vi "control_Indication.vi"(7 "Параметры":T1, 8 "Error In":errorcluster, 9 "control_Pair ref in":refnum<vi>, 10 "control_Port_2 ref in":refnum<vi>, 11 "control_Port_1 ref in":refnum<vi>) -> (0 "Error Out":errorcluster, 1 "control_Pair ref out":refnum<vi>, 2 "control_Port_2 ref out":refnum<vi>, 3 "control_Port_1 ref out":refnum<vi>)   [LabVIEW 2023, in "pump_Lib.lvlib"]
uses:
  pump_Lib.lvlib
  TypeDef/pump_Type.ctl
  TypeDef/pair_Type.ctl
  TypeDef/parametrs_Type.ctl
panel:
  # "%"
  # "%"
  # "%"
  # "%"
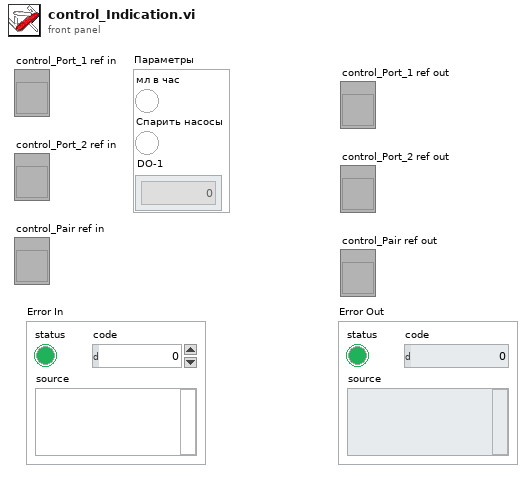
[diagram p1: front panel]
types:
  T1 = typedef "pump_Lib.lvlib/parametrs_Type.ctl" = cluster{"мл в час":bool, "Спарить насосы":bool, "DO-1":u16[]}
  T2 = enum8{"Enabled", "Disabled", "Disabled and Grayed Out"}
  T3 = typedef "pump_Lib.lvlib/pump_Type.ctl" = cluster{"Давление заданное":dbl, "Давление MAX заданное":dbl, "Давление в насосе":dbl, "Давление в системе":dbl, "Расход заданый":dbl, "Расход текущий":dbl, "Объём заданный":dbl, "Объём текущий":dbl, "Позиция насоса %":dbl, "Ток двигателя":dbl, "controlMsg":string, "Клапан k_sys":bool, "Клапан k_res":bool, "Клапан k_air":bool, "Вверх":bool, "Домой":bool, "Вниз":bool, "Старт расход":bool, "Старт давление":bool, "Сброс объёма":bool, "Сброс давления Рсис":bool, "Сброс давления Рнас":bool, "Bits":cluster{"plc_control":bool, "lag_control":bool, "mstop_control":bool, "st_home":bool, "error":bool, "mstart":bool, "pair":bool, "startQ":bool, "startP":bool, "volume_Stop":bool}}
  T4 = typedef "pump_Lib.lvlib/pair_Type.ctl" = cluster{"Давление заданное":dbl, "Давление в системе":dbl, "Расход заданый":dbl, "Расход текущий":dbl, "Объём заданный":dbl, "Объём текущий":dbl, "Старт давление":bool, "Старт расход":bool, "Сброс объёма":bool, "plc_control":bool, "lag_control":bool, "mstop_control":bool, "Давление":cluster{"АЦП CH 0":dbl, "АЦП CH 1":dbl, "АЦП CH 2":dbl, "АЦП CH 3":dbl, "АЦП CH 4":dbl, "АЦП CH 5":dbl, "АЦП CH 6":dbl, "АЦП CH 7":dbl}, "Modbus":cluster{"Массив чтения":u16[], "Массив записи":u16[]}}
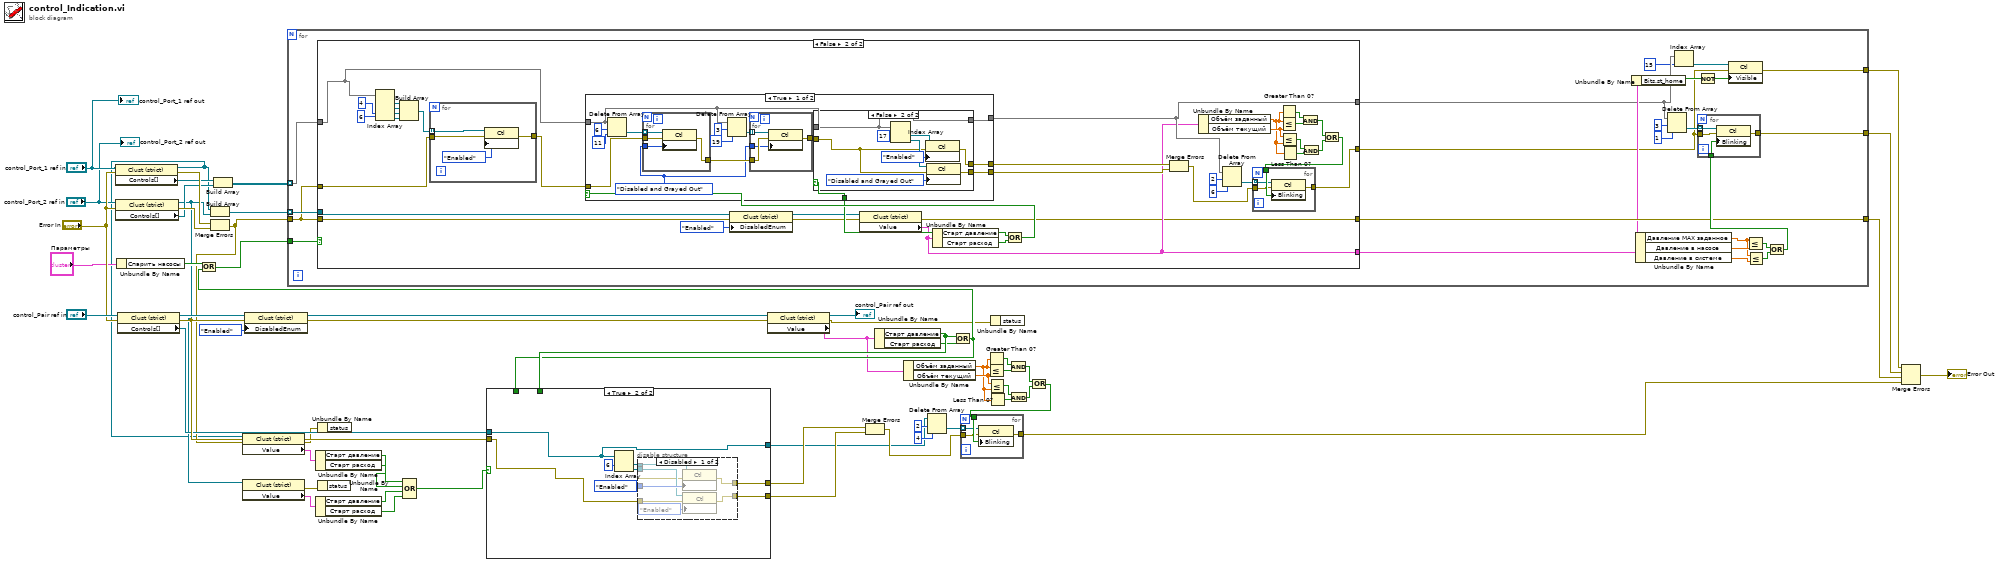
[diagram p0: block diagram]
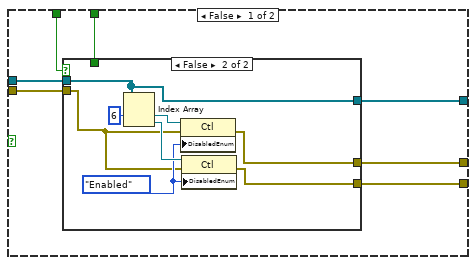
[diagram p2: hidden frame]
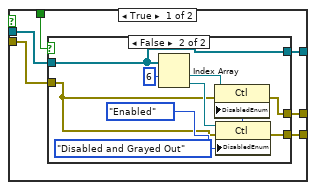
[diagram p3: hidden frame]
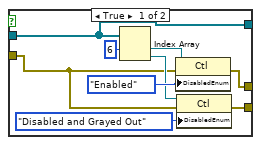
[diagram p4: hidden frame]
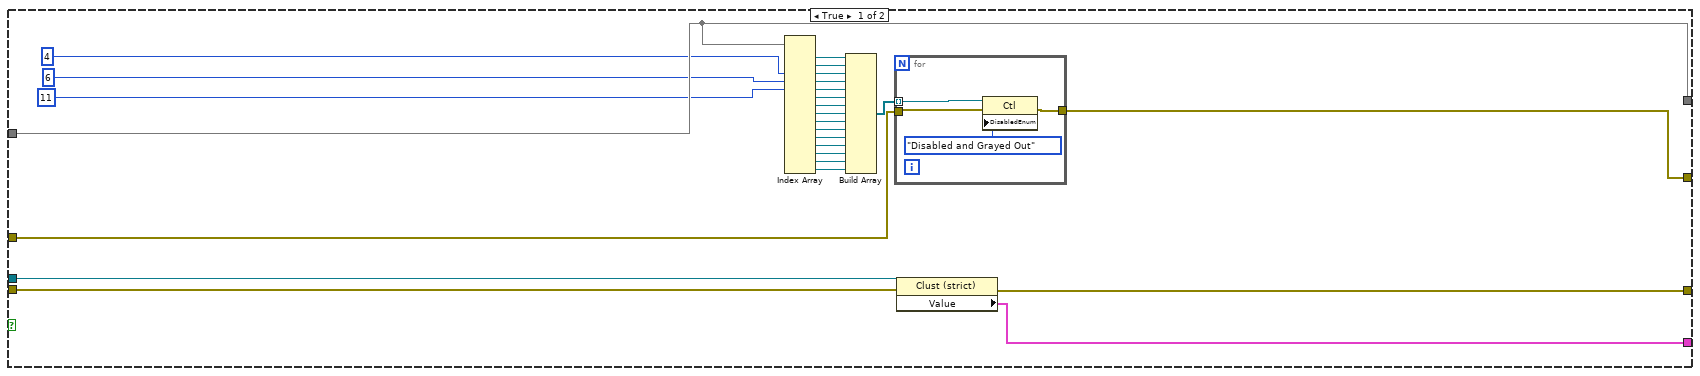
[diagram p6: hidden frame]
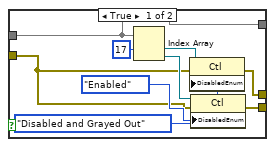
[diagram p7: hidden frame]
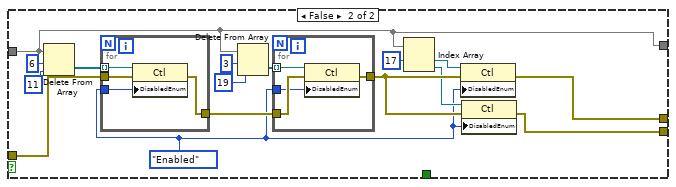
[diagram p8: hidden frame]
diagram:
  n1 = property class="Clust (strict)"(reference="control_Port_1 ref in", error in="Error In") -> (reference out=w11:refnum<vi>, error out=w55:errorcluster, "Controls[]"=w52:refnum<vi>[])
  n2 = property class="Clust (strict)"(reference="control_Port_2 ref in", error in="Error In") -> (reference out=w12:refnum<vi>, error out=w54:errorcluster, "Controls[]"=w51:refnum<vi>[])
  n3 = Unbundle By Name("Параметры") -> ("Спарить насосы"=w41:bool)
  n4 = property class="Clust (strict)"(reference="control_Pair ref in", error in="Error In") -> (reference out=w45:refnum<vi>, error out=w44:errorcluster, "Controls[]"=w43:refnum<vi>[])
  n5 = Build Array(w11, w12) -> (w53:refnum<vi>[])
  n6 = Merge Errors(w55, w54) -> (w13:errorcluster)
  n7 = Build Array(w52, w51) -> (w56:refnum<vi>[][])
  n8 = property class="Clust (strict)"(reference=w11, error in=w13) -> (error out=w8:errorcluster, "Value"=w10:T3)  [unwired: 1 out]
  n9 = property class="Clust (strict)"(reference=w12) -> (error out=w7:errorcluster, "Value"=w9:T3)  [unwired: 1 in, 1 out]
  n10 = property class="Clust (strict)"(reference=w45, error in=w44, "DisabledEnum"=T2."Enabled" ("Disabled")) -> (reference out=w47:refnum<vi>, error out=w48:errorcluster)
  n11 = Unbundle By Name(w10) -> ("Старт давление"=w6:bool, "Старт расход"=w5:bool)
  n12 = Unbundle By Name(w9) -> ("Старт давление"=w4:bool, "Старт расход"=w3:bool)
  n13 = Unbundle By Name(w7) -> ()  [unwired: 1 out]
  n14 = Unbundle By Name(w8) -> ()  [unwired: 1 out]
  n15 = Compound Arithmetic op=OR(w6, w5, w4, w3) -> (w2:bool)
  n16 = property class="Clust (strict)"(reference=w47, error in=w48) -> (reference out=→"control_Pair ref out":refnum<vi>, error out=w1:errorcluster, "Value"=w30:T4)
  n17 = Unbundle By Name(w30) -> ("Старт давление"=w50:bool, "Старт расход"=w49:bool)
  n18 = Unbundle By Name(w30) -> ("Объём заданный"=w26:dbl, "Объём текущий"=w27:dbl)
  n19 = Or(x=w50, y=w49) -> (x .or. y?=w39:bool)
  n20 = Or(x=w41, y=w39) -> (x .or. y?=w40:bool)
  n21 = for {
    tunnel: w56 -> [w81] mode=indexing
    tunnel: w53 -> [w80] mode=indexing
    tunnel: w13 -> [w79]
    tunnel: w40 -> [w78]
    tunnel: [w68] -> w16
    tunnel: [w67] -> w17
    tunnel: [w60] -> w14
    n22 = case shown="False" w78 {
      tunnel: w81 -> [w107 w130]
      tunnel: w79 -> [w87 w128]
      tunnel: w80 -> [w110 w118]
      tunnel: w79 -> [w111 w117]
      tunnel: [w107 w134] -> w64
      tunnel: [w86 w133] -> w61
      tunnel: [w109 w132] -> w66
      tunnel: [w108 w131] -> w68
      frame True {
        n23 = Index Array(array=w107, index #3=4 ("index"), index #4=6 ("index"), index #5=11 ("index")) -> (element #1=w103:refnum<vi>, element #2=w102:refnum<vi>, element #3=w101:refnum<vi>, element #4=w100:refnum<vi>, element #5=w99:refnum<vi>, element #6=w98:refnum<vi>, element #7=w97:refnum<vi>, element #8=w95:refnum<vi>, element #9=w96:refnum<vi>, element #10=w94:refnum<vi>, element #11=w93:refnum<vi>, element #12=w92:refnum<vi>, element #13=w91:refnum<vi>, element #14=w90:refnum<vi>, element #15=w89:refnum<vi>)  [unwired: 12 in]
        n24 = Build Array(w103, w102, w101, w100, w99, w98, w97, w95, w96, w94, w93, w92, w91, w90, w89) -> (w88:refnum<vi>[])
        n25 = for {
          tunnel: w88 -> [w115] mode=indexing
          tunnel: w87 -> [w114]
          tunnel: [w113] -> w86
          n26 = property class="Ctl"(reference=w115, error in=w114, "DisabledEnum"=T2."Disabled and Grayed Out" ("Disabled")) -> (error out=w113:errorcluster)  [unwired: 1 out]
        }
        n27 = property class="Clust (strict)"(reference=w110, error in=w111) -> (error out=w108:errorcluster, "Value"=w109:T3)  [unwired: 1 out]
      }
      frame False {
        n28 = Index Array(array=w130, index #3=4 ("index"), index #4=6 ("index")) -> (element #1=w123:refnum<vi>, element #2=w124:refnum<vi>, element #3=w125:refnum<vi>, element #4=w126:refnum<vi>)  [unwired: 2 in]
        n29 = Build Array(w123, w124, w125, w126) -> (w127:refnum<vi>[])
        n30 = for {
          tunnel: w127 -> [w156] mode=indexing
          tunnel: w128 -> [w155]
          tunnel: [w154] -> w129
          n31 = property class="Ctl"(reference=w156, error in=w155, "DisabledEnum"=T2."Enabled" ("Disabled")) -> (error out=w154:errorcluster)  [unwired: 1 out]
        }
        n32 = property class="Clust (strict)"(reference=w118, error in=w117, "DisabledEnum"=T2."Enabled" ("Disabled")) -> (reference out=w119:refnum<vi>, error out=w120:errorcluster)
        n33 = property class="Clust (strict)"(reference=w119, error in=w120) -> (error out=w131:errorcluster, "Value"=w132:T3)  [unwired: 1 out]
        n34 = Unbundle By Name(w132) -> ("Старт давление"=w150:bool, "Старт расход"=w152:bool)
        n35 = Or(x=w150, y=w152) -> (x .or. y?=w151:bool)
        n36 = case shown="True" w151 {
          tunnel: w129 -> [w172 w214]
          tunnel: w130 -> [w165 w204]
          tunnel: [w164 w204] -> w134
          tunnel: w150 -> [w163 _]
          tunnel: [w162 w203] -> w137
          tunnel: [w161 w202] -> w136
          frame True {
            w167 = T2."Disabled and Grayed Out" ("Disabled")
            n37 = Delete From Array(array=w165, length=6, index=11) -> (deleted portion=w173:refnum<vi>[])  [unwired: 1 out]
            n38 = for {
              tunnel: w173 -> [w201] mode=indexing
              tunnel: w172 -> [w200]
              tunnel: w167 -> [w199]
              tunnel: [w198] -> w168
              n39 = property class="Ctl"(reference=w201, error in=w200, "DisabledEnum"=w199) -> (error out=w198:errorcluster)  [unwired: 1 out]
            }
            n40 = Delete From Array(array=w165, length=3, index=19) -> (deleted portion=w169:refnum<vi>[])  [unwired: 1 out]
            n41 = for {
              tunnel: w169 -> [w197] mode=indexing
              tunnel: w168 -> [w196]
              tunnel: w167 -> [w195]
              tunnel: [w194] -> w166
              n42 = property class="Ctl"(reference=w197, error in=w196, "DisabledEnum"=w195) -> (error out=w194:errorcluster)  [unwired: 1 out]
            }
            n43 = case shown="False" w163 {
              tunnel: w165 -> [w179 w187]
              tunnel: [w179 w187] -> w164
              tunnel: w166 -> [w178 w188]
              tunnel: [w177 w186] -> w162
              tunnel: [w176 w185] -> w161
              frame True {
                n44 = Index Array(array=w179, index #1=17 ("index")) -> (element #1=w183:refnum<vi>, element #2=w182:refnum<vi>)  [unwired: 1 in]
                n45 = property class="Ctl"(reference=w183, error in=w178, "DisabledEnum"=T2."Disabled and Grayed Out" ("Disabled")) -> (error out=w177:errorcluster)  [unwired: 1 out]
                n46 = property class="Ctl"(reference=w182, error in=w178, "DisabledEnum"=T2."Enabled" ("Disabled")) -> (error out=w176:errorcluster)  [unwired: 1 out]
              }
              frame False {
                n47 = Index Array(array=w187, index #1=17 ("index")) -> (element #1=w191:refnum<vi>, element #2=w189:refnum<vi>)  [unwired: 1 in]
                n48 = property class="Ctl"(reference=w191, error in=w188, "DisabledEnum"=T2."Enabled" ("Disabled")) -> (error out=w186:errorcluster)  [unwired: 1 out]
                n49 = property class="Ctl"(reference=w189, error in=w188, "DisabledEnum"=T2."Disabled and Grayed Out" ("Disabled")) -> (error out=w185:errorcluster)  [unwired: 1 out]
              }
            }
          }
          frame False {
            w205 = T2."Enabled" ("Disabled")
            n50 = Delete From Array(array=w204, length=6, index=11) -> (deleted portion=w215:refnum<vi>[])  [unwired: 1 out]
            n51 = for {
              tunnel: w215 -> [w225] mode=indexing
              tunnel: w214 -> [w224]
              tunnel: w205 -> [w223]
              tunnel: [w222] -> w210
              n52 = property class="Ctl"(reference=w225, error in=w224, "DisabledEnum"=w223) -> (error out=w222:errorcluster)  [unwired: 1 out]
            }
            n53 = Delete From Array(array=w204, length=3, index=19) -> (deleted portion=w211:refnum<vi>[])  [unwired: 1 out]
            n54 = for {
              tunnel: w211 -> [w221] mode=indexing
              tunnel: w210 -> [w220]
              tunnel: w205 -> [w219]
              tunnel: [w218] -> w209
              n55 = property class="Ctl"(reference=w221, error in=w220, "DisabledEnum"=w219) -> (error out=w218:errorcluster)  [unwired: 1 out]
            }
            n56 = Index Array(array=w204, index #1=17 ("index")) -> (element #1=w207:refnum<vi>, element #2=w206:refnum<vi>)  [unwired: 1 in]
            n57 = property class="Ctl"(reference=w207, error in=w209, "DisabledEnum"=w205) -> (error out=w203:errorcluster)  [unwired: 1 out]
            n58 = property class="Ctl"(reference=w206, error in=w209, "DisabledEnum"=w205) -> (error out=w202:errorcluster)  [unwired: 1 out]
          }
        }
        n59 = Merge Errors(w137, w136) -> (w135:errorcluster)
        n60 = Unbundle By Name(w132) -> ("Объём заданный"=w143:dbl, "Объём текущий"=w144:dbl)
        n61 = Delete From Array(array=w134, length=2, index=6) -> (deleted portion=w147:refnum<vi>[])  [unwired: 1 out]
        n62 = Greater Than 0?(x=w143) -> (x > 0?=w145:bool)
        n63 = Less Or Equal?(x=w143, y=w144) -> (x <= y?=w146:bool)
        n64 = Less Or Equal?(x=w144, y=w143) -> (x <= y?=w141:bool)
        n65 = Less Than 0?(x=w143) -> (x < 0?=w142:bool)
        n66 = And(x=w145, y=w146) -> (x .and. y?=w140:bool)
        n67 = And(x=w141, y=w142) -> (x .and. y?=w139:bool)
        n68 = Or(x=w140, y=w139) -> (x .or. y?=w138:bool)
        n69 = for {
          tunnel: w138 -> [w160]
          tunnel: w147 -> [w159] mode=indexing
          tunnel: w135 -> [w158]
          tunnel: [w157] -> w133
          n70 = property class="Ctl"(reference=w159, error in=w158, "Blinking"=w160) -> (error out=w157:errorcluster)  [unwired: 1 out]
        }
      }
    }
    n71 = Unbundle By Name(w66) -> ("Bits.st_home"=w65:bool)
    n72 = Unbundle By Name(w66) -> ("Давление MAX заданное"=w73:dbl, "Давление в насосе"=w74:dbl, "Давление в системе"=w72:dbl)
    n73 = Delete From Array(array=w64, length=3, index=1) -> (deleted portion=w77:refnum<vi>[])  [unwired: 1 out]
    n74 = Index Array(array=w64, index=15) -> (element=w63:refnum<vi>)
    n75 = Not(x=w65) -> (.not. x?=w59:bool)
    n76 = property class="Ctl"(reference=w63, error in=w61, "Visible"=w59) -> (error out=w60:errorcluster)  [unwired: 1 out]
    n77 = Less Or Equal?(x=w73, y=w74) -> (x <= y?=w71:bool)
    n78 = Less Or Equal?(x=w73, y=w72) -> (x <= y?=w70:bool)
    n79 = Or(x=w71, y=w70) -> (x .or. y?=w69:bool)
    n80 = for {
      tunnel: w77 -> [w83] mode=indexing
      tunnel: [w85] -> w67
      tunnel: w61 -> [w84]
      tunnel: w69 -> [w82]
      n81 = property class="Ctl"(reference=w83, error in=w84, "Blinking"=w82) -> (error out=w85:errorcluster)  [unwired: 1 out]
    }
  }
  n82 = case shown="True" w2 {
    tunnel: w50 -> [w232 _]
    tunnel: w44 -> [w231 w267]
    tunnel: w43 -> [w230 w268]
    tunnel: w39 -> [w229 _]
    tunnel: [w228 w266] -> w33
    tunnel: [w227 w265] -> w32
    tunnel: [w226 w268] -> w19
    frame False {
      n83 = case shown="False" w229 {
        tunnel: w231 -> [w236 w260]
        tunnel: w230 -> [w238 w259]
        tunnel: [w237 w259] -> w226
        tunnel: w232 -> [w235 _]
        tunnel: [w234 w258] -> w228
        tunnel: [w233 w257] -> w227
        frame True {
          n84 = case shown="False" w235 {
            tunnel: w238 -> [w241 w251]
            tunnel: [w241 w251] -> w237
            tunnel: w236 -> [w242 w250]
            tunnel: [w240 w249] -> w234
            tunnel: [w239 w248] -> w233
            frame True {
              n85 = Index Array(array=w241, index #1=6 ("index")) -> (element #1=w245:refnum<vi>, element #2=w243:refnum<vi>)  [unwired: 1 in]
              n86 = property class="Ctl"(reference=w245, error in=w242, "DisabledEnum"=T2."Enabled" ("Disabled")) -> (error out=w240:errorcluster)  [unwired: 1 out]
              n87 = property class="Ctl"(reference=w243, error in=w242, "DisabledEnum"=T2."Disabled and Grayed Out" ("Disabled")) -> (error out=w239:errorcluster)  [unwired: 1 out]
            }
            frame False {
              n88 = Index Array(array=w251, index #1=6 ("index")) -> (element #1=w255:refnum<vi>, element #2=w254:refnum<vi>)  [unwired: 1 in]
              n89 = property class="Ctl"(reference=w255, error in=w250, "DisabledEnum"=T2."Disabled and Grayed Out" ("Disabled")) -> (error out=w249:errorcluster)  [unwired: 1 out]
              n90 = property class="Ctl"(reference=w254, error in=w250, "DisabledEnum"=T2."Enabled" ("Disabled")) -> (error out=w248:errorcluster)  [unwired: 1 out]
            }
          }
        }
        frame False {
          w261 = T2."Enabled" ("Disabled")
          n91 = Index Array(array=w259, index #1=6 ("index")) -> (element #1=w263:refnum<vi>, element #2=w262:refnum<vi>)  [unwired: 1 in]
          n92 = property class="Ctl"(reference=w263, error in=w260, "DisabledEnum"=w261) -> (error out=w258:errorcluster)  [unwired: 1 out]
          n93 = property class="Ctl"(reference=w262, error in=w260, "DisabledEnum"=w261) -> (error out=w257:errorcluster)  [unwired: 1 out]
        }
      }
    }
    frame True {
      n94 = Index Array(array=w268, index #1=6 ("index")) -> (element #1=w270:refnum<vi>, element #2=w269:refnum<vi>)  [unwired: 1 in]
      n95 = disable-structure shown="Disabled" {
        disable-tunnel: T2."Enabled" ("Disabled") -> [w279 _]
        disable-tunnel: w270 -> [w278 _]
        disable-tunnel: w269 -> [w276 _]
        disable-tunnel: w267 -> [w275 _]
        disable-tunnel: [w274 _] -> w266
        disable-tunnel: [w273 _] -> w265
        frame Disabled {
          n96 = property class="Ctl"(reference=w278, error in=w275, "DisabledEnum"=w279) -> (error out=w274:errorcluster)  [unwired: 1 out]
          n97 = property class="Ctl"(reference=w276, error in=w275, "DisabledEnum"=T2."Enabled" ("Disabled")) -> (error out=w273:errorcluster)  [unwired: 1 out]
        }
        frame Enabled {
        }
      }
    }
  }
  n98 = Merge Errors(w33, w32) -> (w20:errorcluster)
  n99 = Delete From Array(array=w19, length=2, index=4) -> (deleted portion=w31:refnum<vi>[])  [unwired: 1 out]
  n100 = Greater Than 0?(x=w26) -> (x > 0?=w28:bool)
  n101 = Less Or Equal?(x=w26, y=w27) -> (x <= y?=w29:bool)
  n102 = Less Or Equal?(x=w27, y=w26) -> (x <= y?=w24:bool)
  n103 = Less Than 0?(x=w26) -> (x < 0?=w25:bool)
  n104 = Unbundle By Name(w1) -> ()  [unwired: 1 out]
  n105 = And(x=w28, y=w29) -> (x .and. y?=w23:bool)
  n106 = And(x=w24, y=w25) -> (x .and. y?=w22:bool)
  n107 = Or(x=w23, y=w22) -> (x .or. y?=w21:bool)
  n108 = for {
    tunnel: w21 -> [w283]
    tunnel: w31 -> [w282] mode=indexing
    tunnel: w20 -> [w281]
    tunnel: [w280] -> w15
    n109 = property class="Ctl"(reference=w282, error in=w281, "Blinking"=w283) -> (error out=w280:errorcluster)  [unwired: 1 out]
  }
  n110 = Merge Errors(w14, w17, w16, w15) -> (→"Error Out":errorcluster)
  "control_Port_1 ref out" <- "control_Port_1 ref in"
  "control_Port_2 ref out" <- "control_Port_2 ref in"
